vi "remap tag and channel.vi"(7 "instance id":string, 8 "error in":errorcluster, 9 "tag name":string, 10 "channel":refnum<class "TBM channel.lvclass">, 11 "engine configuration in":refnum<class "engine configuration.lvclass">) -> (0 "error out":errorcluster, 3 "engine configuration out":refnum<class "engine configuration.lvclass">)   [LabVIEW 2013, in "Logic Sequencer editor node.lvclass"]
uses:
  Logic Sequencer editor node.lvclass
  <vilib>/NI/Module Execution Interface/Engine Configuration/engine configuration.lvclass
  <vilib>/NI/Tag Bus Module Framework/channel/TBM channel.lvclass
  <vilib>/NI/Tag Bus/tag/tag descriptor.lvclass/tag descriptor.ctl
  <vilib>/NI/Tag Bus/tag/tag descriptor.lvclass
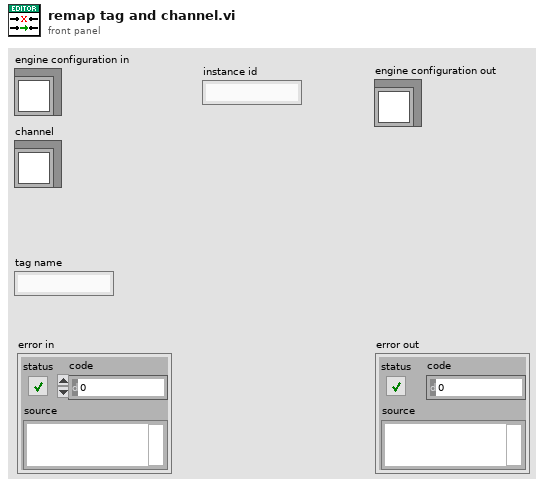
[diagram p1: front panel]
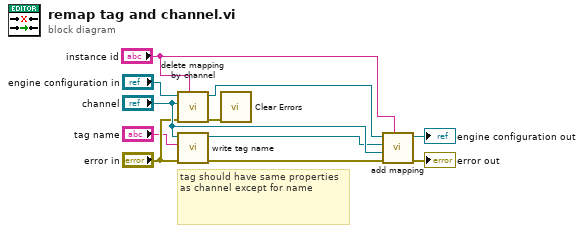
[diagram p0: block diagram]
diagram:
  # "tag should have same properties as channel except for name"
  n1 = call <vilib>:"delete mapping by channel.vi"("owner ID"="instance id", "error in"="error in", "channel"="channel", "engine configuration in"="engine configuration in") -> ("error out"=w11:errorcluster, "engine configuration out"=w4:refnum<class "engine configuration.lvclass">)  [unwired: 6 in]
  n2 = call <vilib>:"write tag name.vi"("error in"="error in", "name"="tag name", "system tag in"="channel") -> ("error out"=w7:errorcluster, "system tag out"=w5:refnum<class "TBM channel.lvclass">)  [unwired: 7 in]
  n3 = call <vilib>:"Clear Errors.vi"("error in (no error)"=w11) -> ()  [unwired: 6 in, 1 out]
  n4 = call <vilib>:"add mapping.vi"("owner ID"="instance id", "error in"=w7, "channel"="channel", "tag descriptor"=w5, "engine configuration"=w4) -> ("error out"=→"error out":errorcluster, "engine configuration out"=→"engine configuration out":refnum<class "engine configuration.lvclass">)  [unwired: 5 in]
